vi "Read Oculus Rift Guidance Index.vi"(8 "error in (no error)":errorcluster, 11 "Vessel in":refnum<class "Vessel.lvclass">) -> (0 "error out":errorcluster, 2 "Oculus Rift Guidance Index":i32, 3 "Vessel out":refnum<class "Vessel.lvclass">)   [LabVIEW 2014, in "Vessel.lvclass"]
uses:
  Vessel.lvclass
  Vessel.lvclass/Vessel.ctl
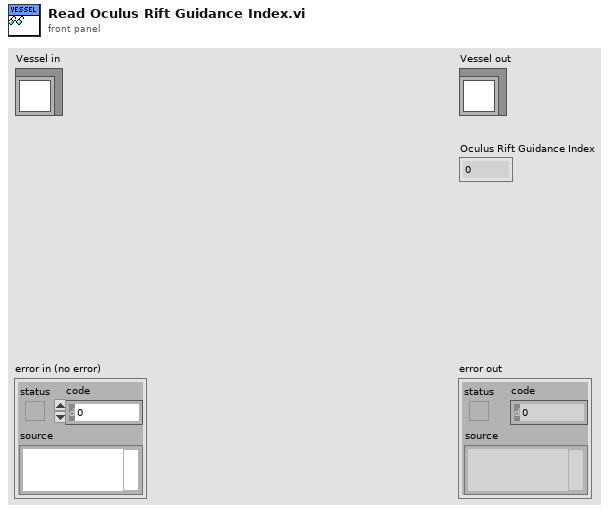
[diagram p1: front panel]
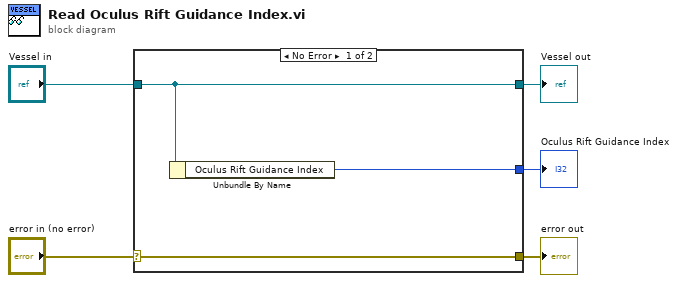
[diagram p0: block diagram]
diagram:
  n1 = case shown="No Error" "error in (no error)" {
    selector: "error in (no error)" -> [w8 w9]
    tunnel: [w8 w9] -> w4
    tunnel: [w7 w10] -> w2
    tunnel: "Vessel in" -> [w7 w10]
    tunnel: [w6 _] -> w1
    frame No Error {
      n2 = Unbundle By Name(w7) -> ("Oculus Rift Guidance Index"=w6:i32)
    }
    frame Error {
    }
  }
  "error out" <- w4
  "Vessel out" <- w2
  "Oculus Rift Guidance Index" <- w1
